vi "Periodic Tasks.vi"(8 "error in":errorcluster) -> ()   [LabVIEW 2014]
doc: "This VI runs in parallel to other tasks. It can contain as many user-defined periodic loops as you need. These can carry out PID or other sorts of timed response."
panel:
  out "Data Out":u8[](array[numeric])
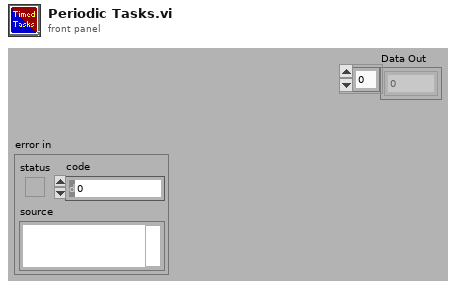
[diagram p1: front panel]
types:
  T1 = typedef "WPI_I2CDevRef.ctl" = cluster{"DevStatus":errorcluster, "Controller":T2, "Device Address":u8, "Handle":i32, "I2C Bus":T3}
  T2 = typedef "FPGA_TypedefDigitalModule.ctl" = enum16{"Controller 1"}
  T3 = typedef "i2c_bus.ctl" = enum16{"I2C On-Board", "I2C MXP", "Invalid"}
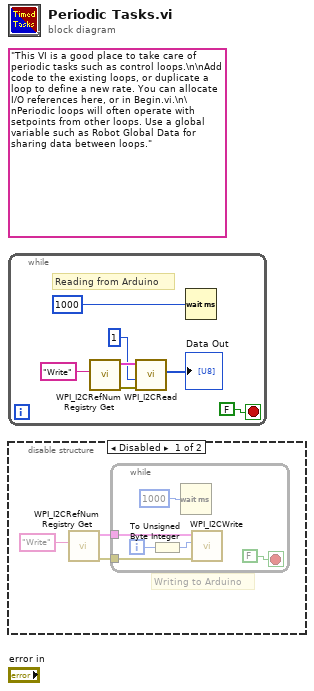
[diagram p0: block diagram]
diagram:
  (unwired) "This VI is a good place to take care of periodic tasks such as control loops.\n\nAdd code to the existing loops, or duplicate a loop to define a new rate. You can allocate I/O references here, or in Begin.vi.\n\nPeriodic loops will often operate with setpoints from other loops. Use a global variable such as Robot Global Data for sharing data between loops."
  n1 = while {
    stop <- FALSE stop-if-true
    # "Reading from Arduino"
    n2 = call <vilib>:"WPI_I2CRefNum Registry Get.vi"("refnum name"="Write") -> ("error out"=w3:errorcluster, "I2CDevRef"=w4:T1)  [unwired: 9 in]
    n3 = call <vilib>:"WPI_I2CRead.vi"("error in (no error)"=w3, "I2CBytesToRead"=u8 1, "I2CDevRef"=w4) -> ("Data Out"=→"Data Out":u8[])  [unwired: 6 in, 2 out]
    n4 = Wait (ms)(milliseconds to wait=u32 1000) -> ()  [unwired: 1 out]
  }
  n5 = disable-structure shown="Disabled" {
    frame Disabled {
      # "Writing to Arduino"
      n6 = call <vilib>:"WPI_I2CRefNum Registry Get.vi"("refnum name"="Write") -> ("error out"=w8:errorcluster, "I2CDevRef"=w9:T1)  [unwired: 9 in]
      n7 = while {
        tunnel: w9 -> [w16]
        tunnel: w8 -> [w15]
        i -> [w12]
        stop <- FALSE stop-if-true
        n8 = To Unsigned Byte Integer(number=w12) -> (unsigned 8bit integer=w11:u8)
        n9 = Wait (ms)(milliseconds to wait=u32 1000) -> ()  [unwired: 1 out]
        n10 = call <vilib>:"WPI_I2CWrite.vi"("error in (no error)"=w15, "I2CRegister"=w11, "I2CDevRef"=w16) -> ()  [unwired: 7 in, 2 out]
      }
    }
    frame Enabled {
    }
  }
